vi "写.vi"(8 "错误输入（无错误）":errorcluster, 9 "数据":string[](array[string]), 10 "起始地址":string, 11 "VISA资源名称":refnum<visa-resource-name>) -> (0 "错误输出":errorcluster, 3 "VISA资源名称输出":refnum<visa-resource-name>)   [LabVIEW 2017]
panel:
  out "连接的字符串":string
  in  "命令码":string="WD"
  in  "节点号":string="00"
  # "@00WD000000010002"
  # "通讯格式说明：\n   发送：\n     读：          起始符        节点号                 命令码        开始字             字数         FCS校验码   终止符\n                        @              00                       RD          0000              0002                \n起始符：必须以@开始\n节点号：默认是00，由DM6648和DM6653指定\n命令码：RD（DM数据区读）\n开始字：0000（个人理解是起始地址）（10进制数据）\n字数：0002（要读取的字的个数）（10进制数据）\nFCS校验码：\n终止符：*CR（由*和回车组成）（一定要组合，一次最多字符长度是131超过之后利用的是分隔符来读取的）\n     写：          起始符        节点号           命令码        开始字        第一个数据（字）  第二个数据（字）      FCS校验码    终止符\n                        @              00                WD          0000              0001                    0010\n起始符：必须以@开始\n节点号：默认是00，由DM6648和DM6653指定\n命令码：WD（DM数据区写）\n开始字：0000（个人理解是起始地址）（10进制数据）\n第一/二个数据（字）：0001/0010（写入的数据1和16）（16进制数据）\nFCS校验码：\n终止符：*CR（由*和回车组成）（一定要组合，一次最多字符长度是131超过之后利用的是分隔符来读取的）"
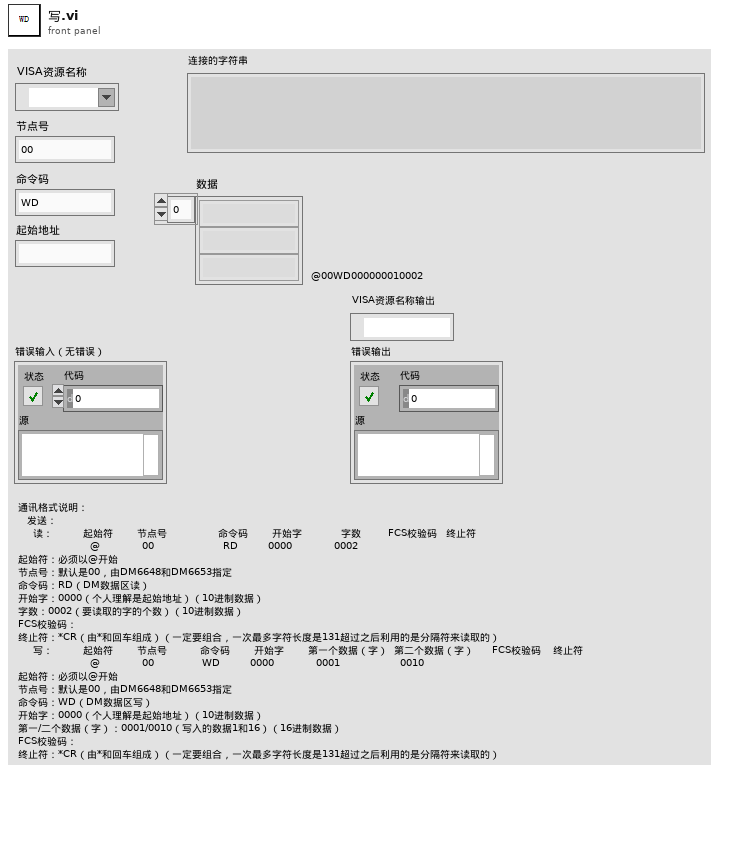
[diagram p1: front panel]
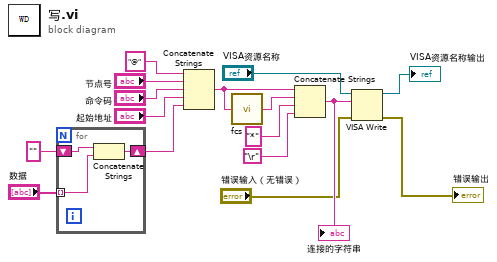
[diagram p0: block diagram]
diagram:
  n1 = for {
    tunnel: "数据" -> [w17] mode=indexing
    shift-right: [w19] -> w4
    shift-left: "" -> [w18]
    n2 = Concatenate Strings(w18, w17) -> (w19:string)
  }
  n3 = Concatenate Strings("@", "节点号", "命令码", "起始地址", w4) -> (w13:string)
  n4 = call "fcs .vi"("string"=w13) -> ("frame check sum"=w12:string)
  n5 = Concatenate Strings(w13, w12, "*" ("搜索字符串"), "\r") -> (w9:string)
  "连接的字符串" <- w9
  n6 = VISA Write(VISA resource name="VISA资源名称", write buffer=w9, error in (no error)="错误输入（无错误）") -> (VISA resource name out=→"VISA资源名称输出":refnum<visa-resource-name>, error out=→"错误输出":errorcluster)  [unwired: 1 out]
